vi "Alphanumeric_keyboard_new.vi"(0 "Str Refnum":refnum<vi>, 1 "Display Style":u32) -> (2 "New String":string, 3 "Previous String":string, 4 "Boolean":bool)   [LabVIEW 2022 SP3]
doc: "This VI takes the control reference for a digital numeric indicator and provides a calculator style keypad for number entry. The reference is double, but it only works for positive, integer values"
uses:
  <vilib>/Utility/miscctls.llb/LVPointTypeDef.ctl
panel:
  in  "SBR":bool
  in  "SBL":bool
  in  "CBR":bool
  in  "CBL":bool
  in  "RBR":bool
  in  "RBL":bool
  in  "Zero":bool
  in  "Percentage":bool
  in  "Space":bool
  in  "Dolor":bool
  in  "Plus":bool
  in  "@":bool
  in  "Under Score":bool
  in  "Has":bool
  in  "Star":bool
  in  "and":bool
  in  "Caps Lock":bool
  in  "Equal":bool
  in  "X":bool
  in  "Z":bool
  in  "C":bool
  in  "Backslash":bool
  in  "Slash":bool
  in  "M":bool
  in  "N":bool
  in  "B":bool
  in  "V":bool
  in  "Minus":bool
  in  "Colon":bool
  in  "S":bool
  in  "D":bool
  in  "A":bool
  in  "Semi Colon":bool
  in  "L":bool
  in  "K":bool
  in  "J":bool
  in  "H":bool
  in  "G":bool
  in  "F":bool
  in  "Comma":bool
  in  "W":bool
  in  "E":bool
  in  "Q":bool
  in  "P":bool
  in  "O":bool
  in  "I":bool
  in  "U":bool
  in  "Y":bool
  in  "T":bool
  in  "R":bool
  in  "Dot":bool
  in  "Enter Text":string
  in  "Enter":bool
  in  "Nine":bool
  in  "Eight":bool
  in  "Seven":bool
  in  "Six":bool
  in  "Five":bool
  in  "Four":bool
  in  "Three":bool
  in  "CLR":bool
  in  "BS":bool
  in  "Cancel":bool
  in  "Two":bool
  in  "One":bool
  out "String":string
  in  "Charactor\nLength":dbl
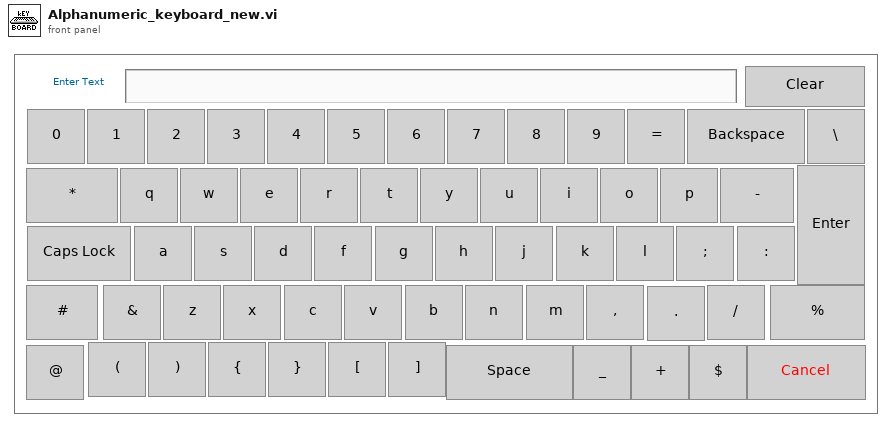
[diagram p1: front panel]
types:
  T1 = typedef "LVPointTypeDef.ctl" = cluster{"Horizontal":i16, "Vertical":i16}
  T2 = enum32{"Invalid", "Default", "Floating", "Floating/Auto-Hide", "Modal"}
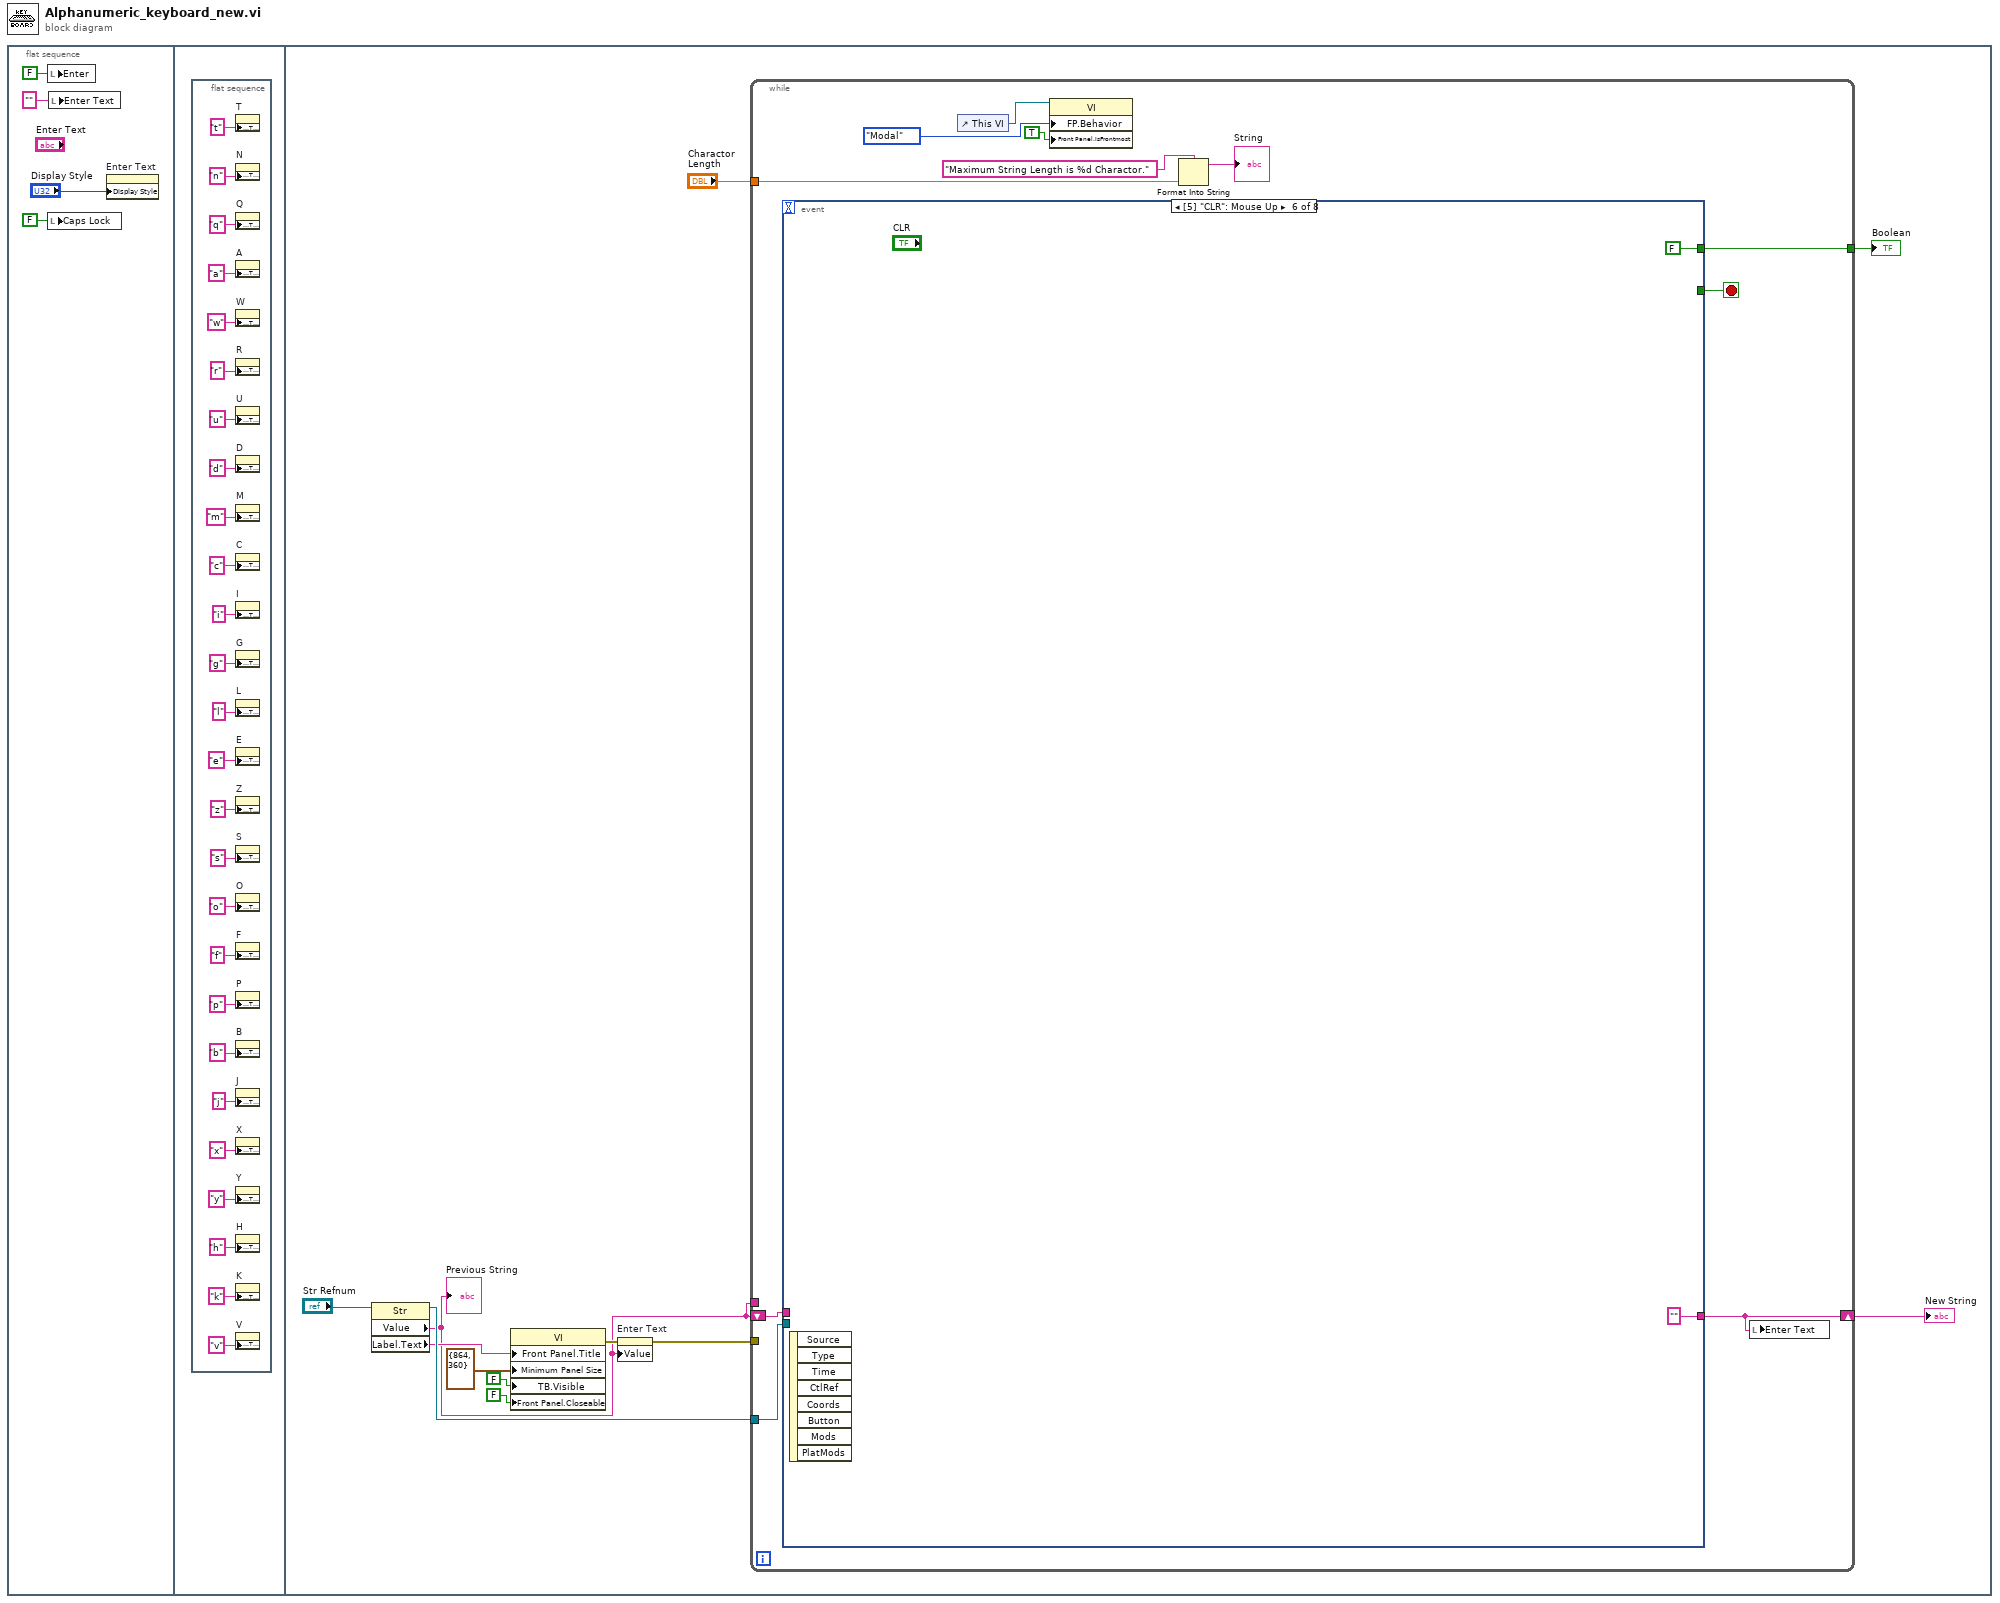
[diagram p0: block diagram]
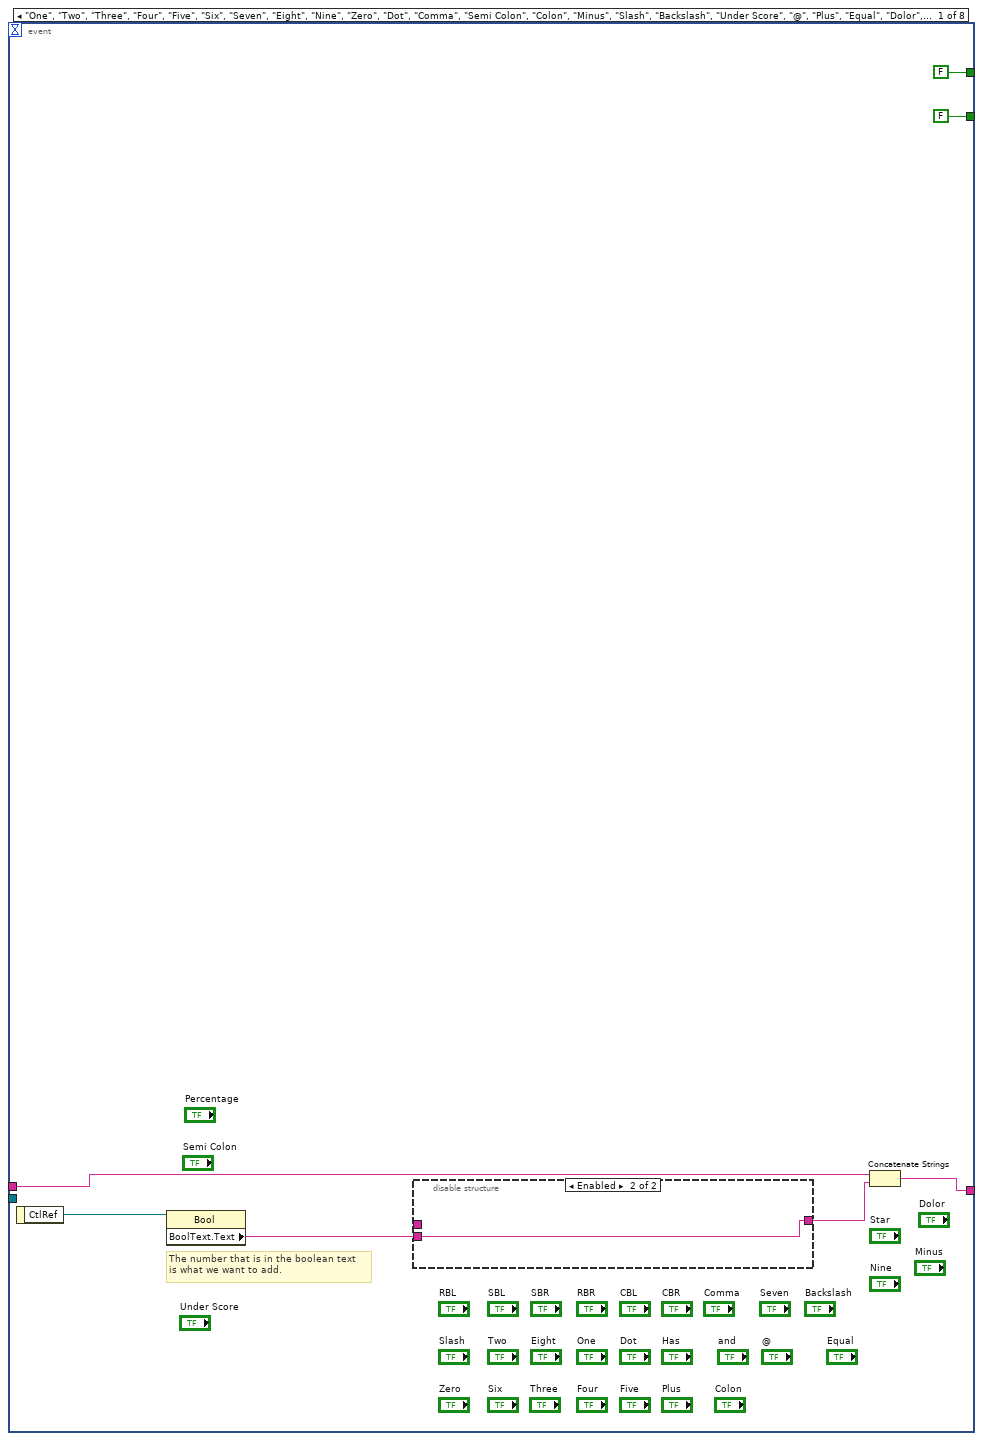
[diagram p2: hidden frame]
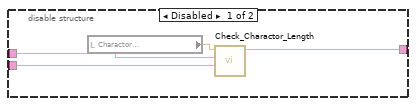
[diagram p3: hidden frame]
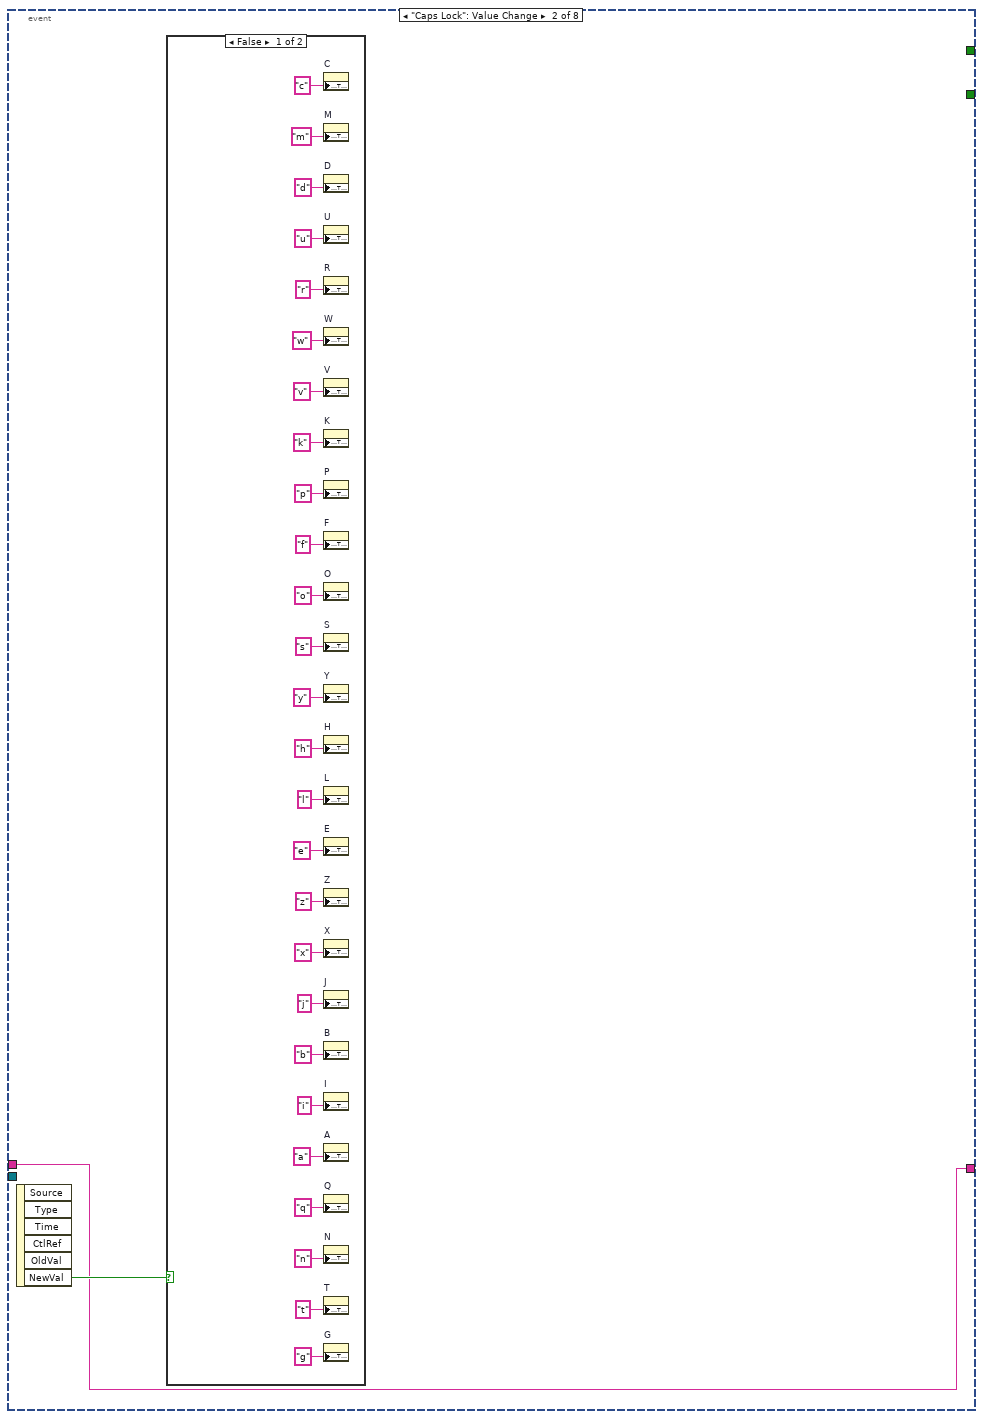
[diagram p4: hidden frame]
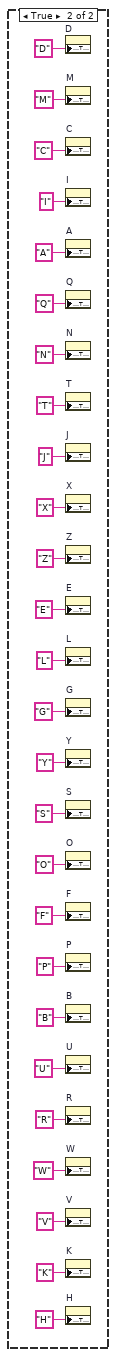
[diagram p5: hidden frame]
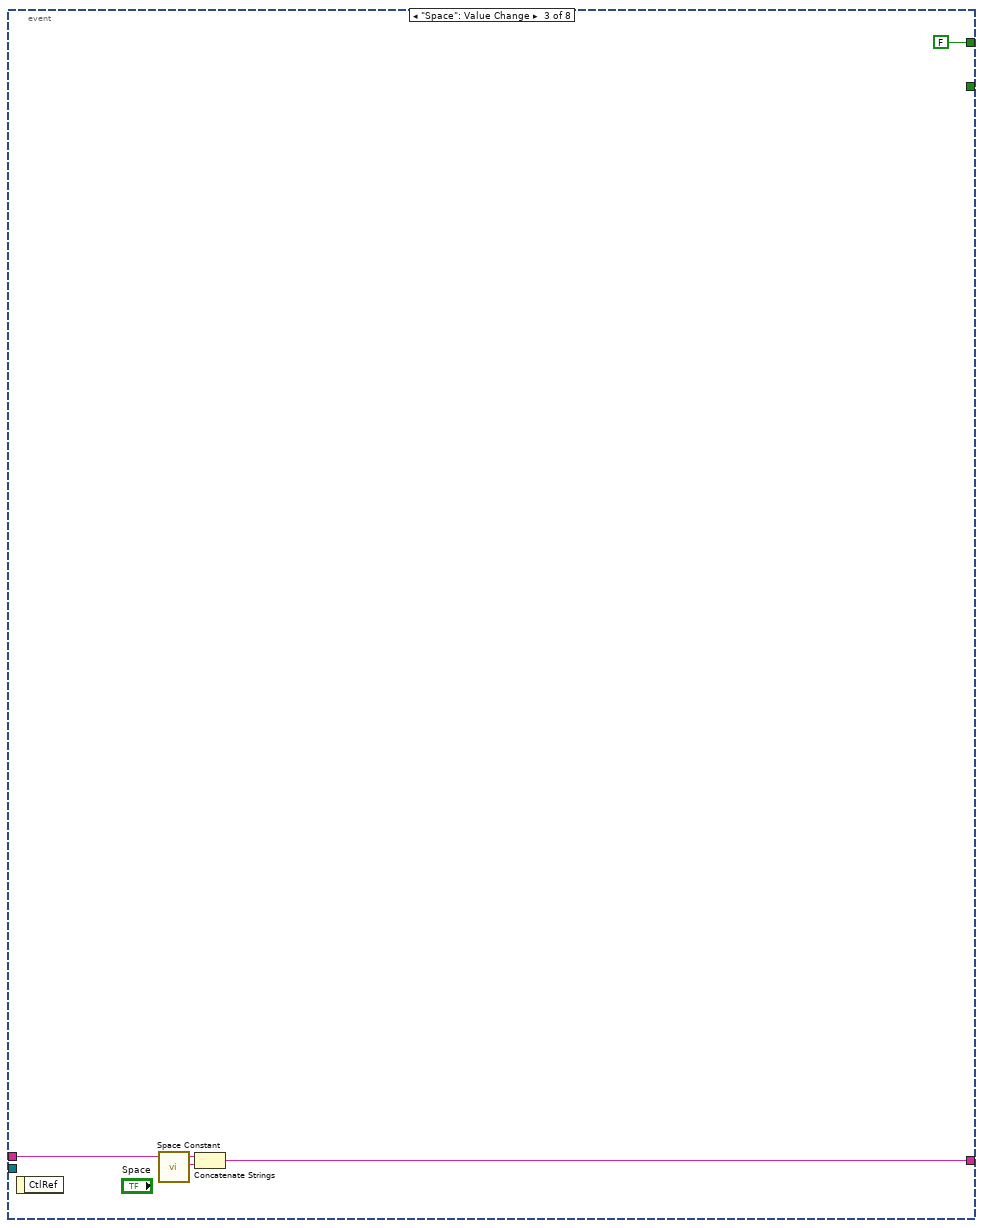
[diagram p6: hidden frame]
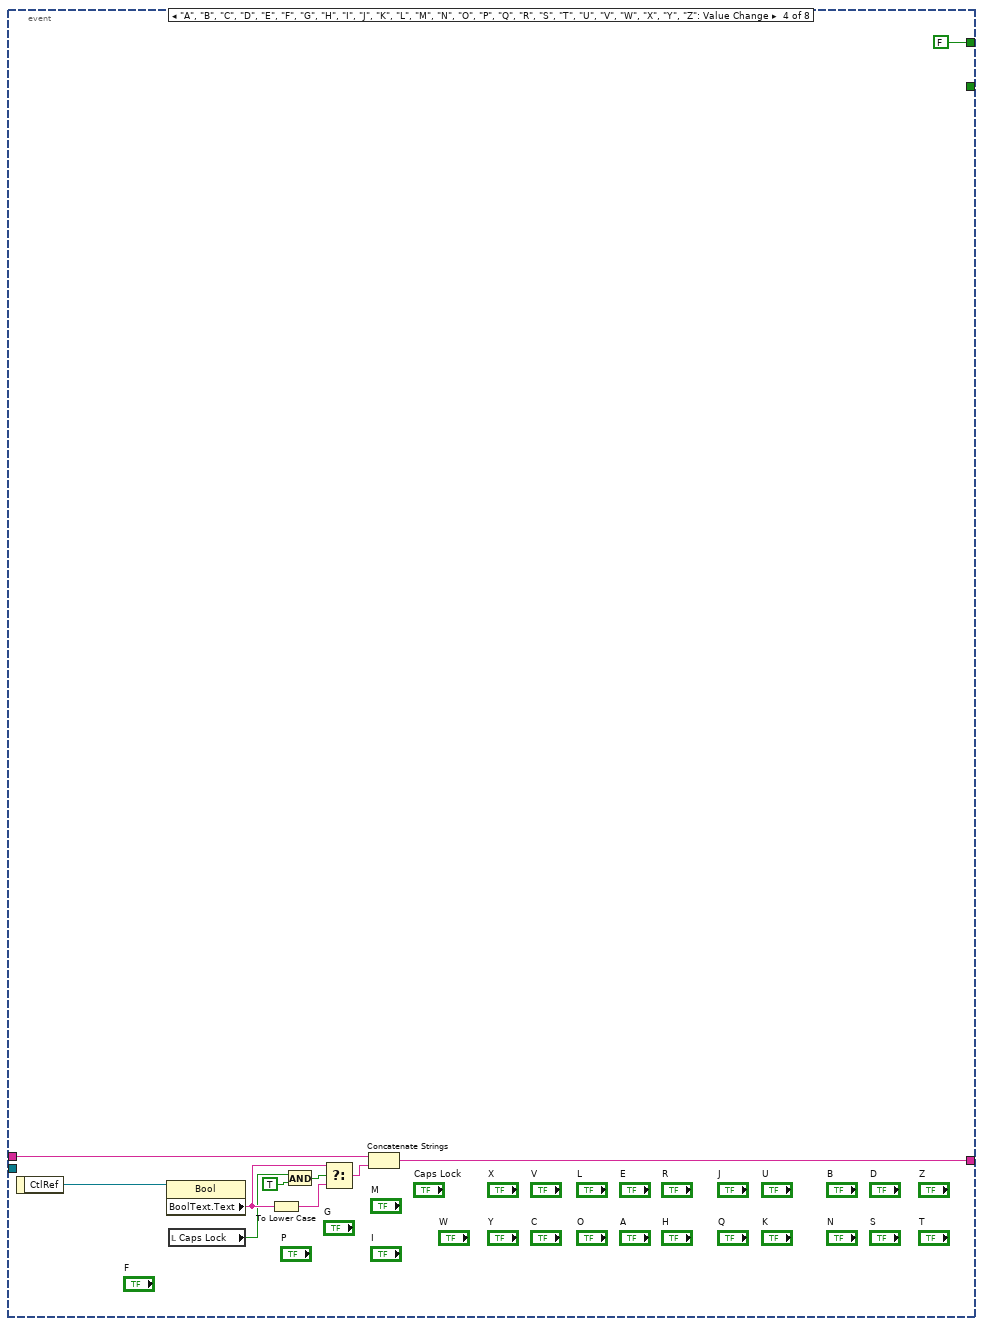
[diagram p7: hidden frame]
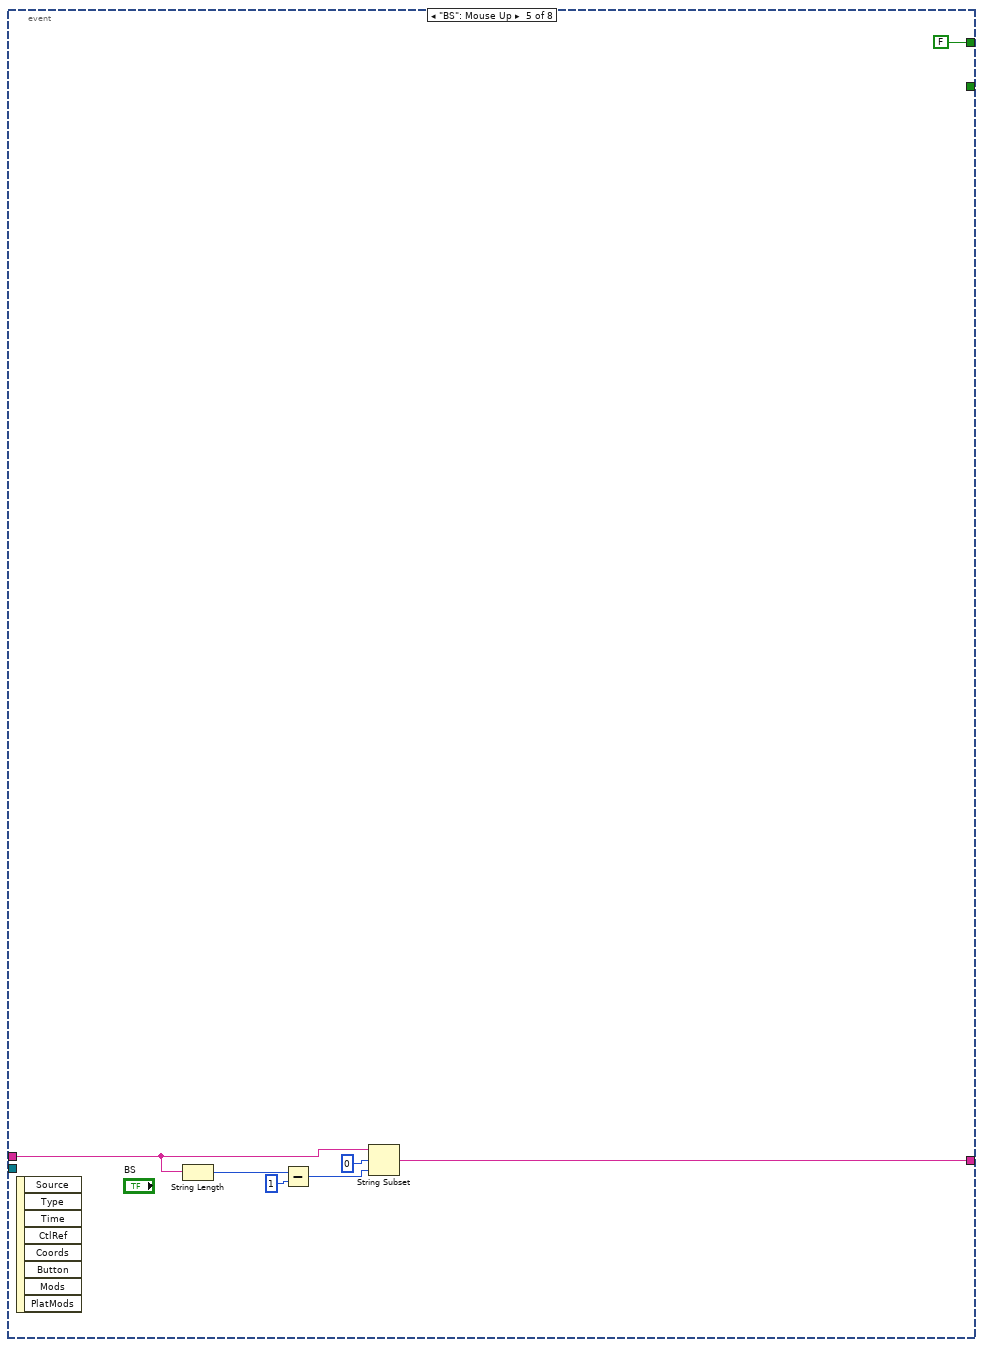
[diagram p8: hidden frame]
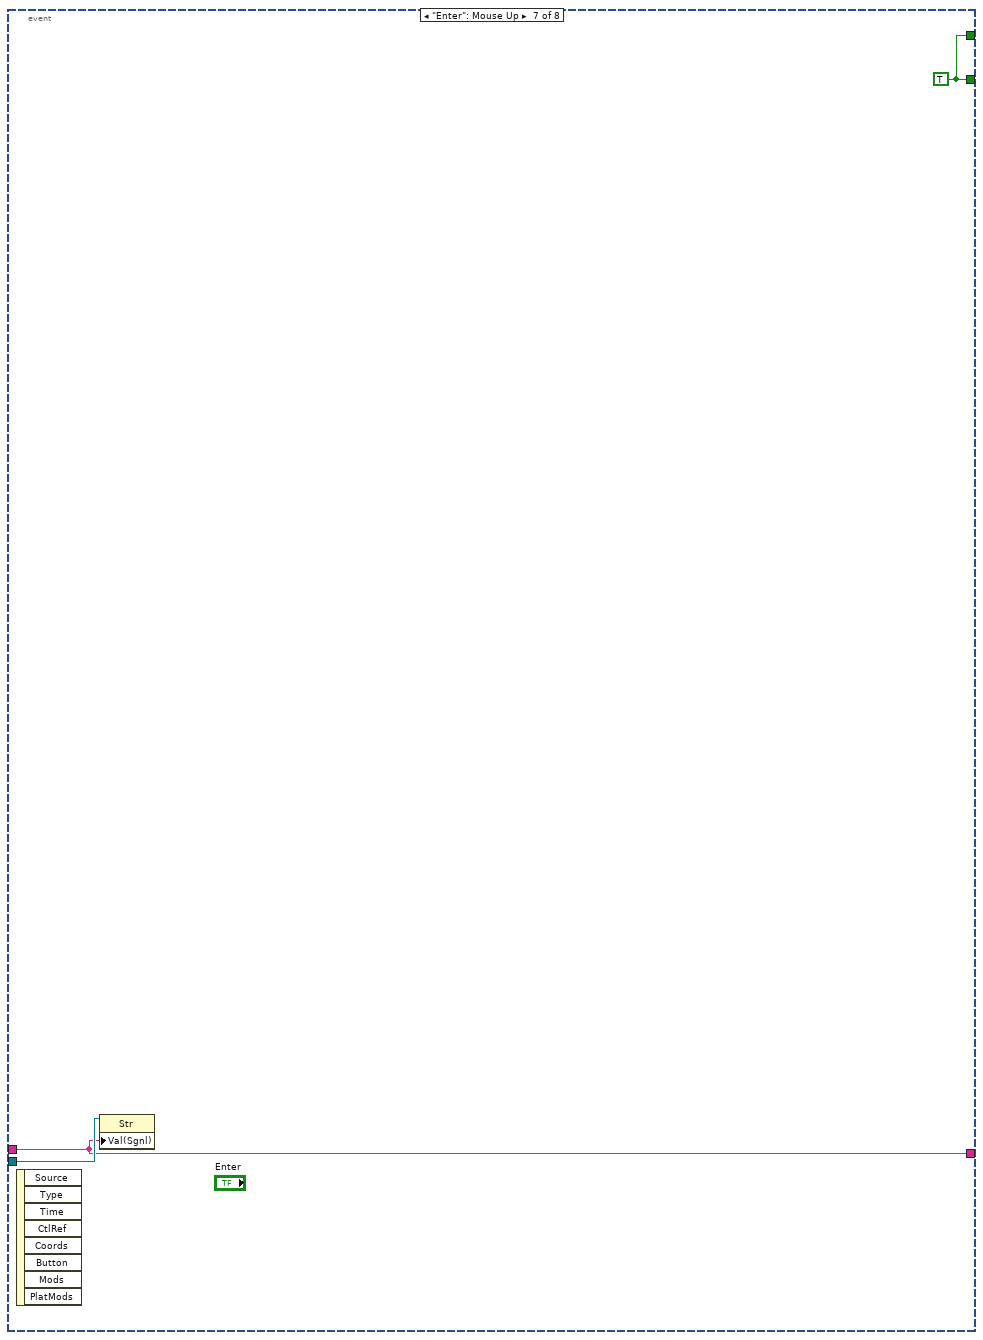
[diagram p9: hidden frame]
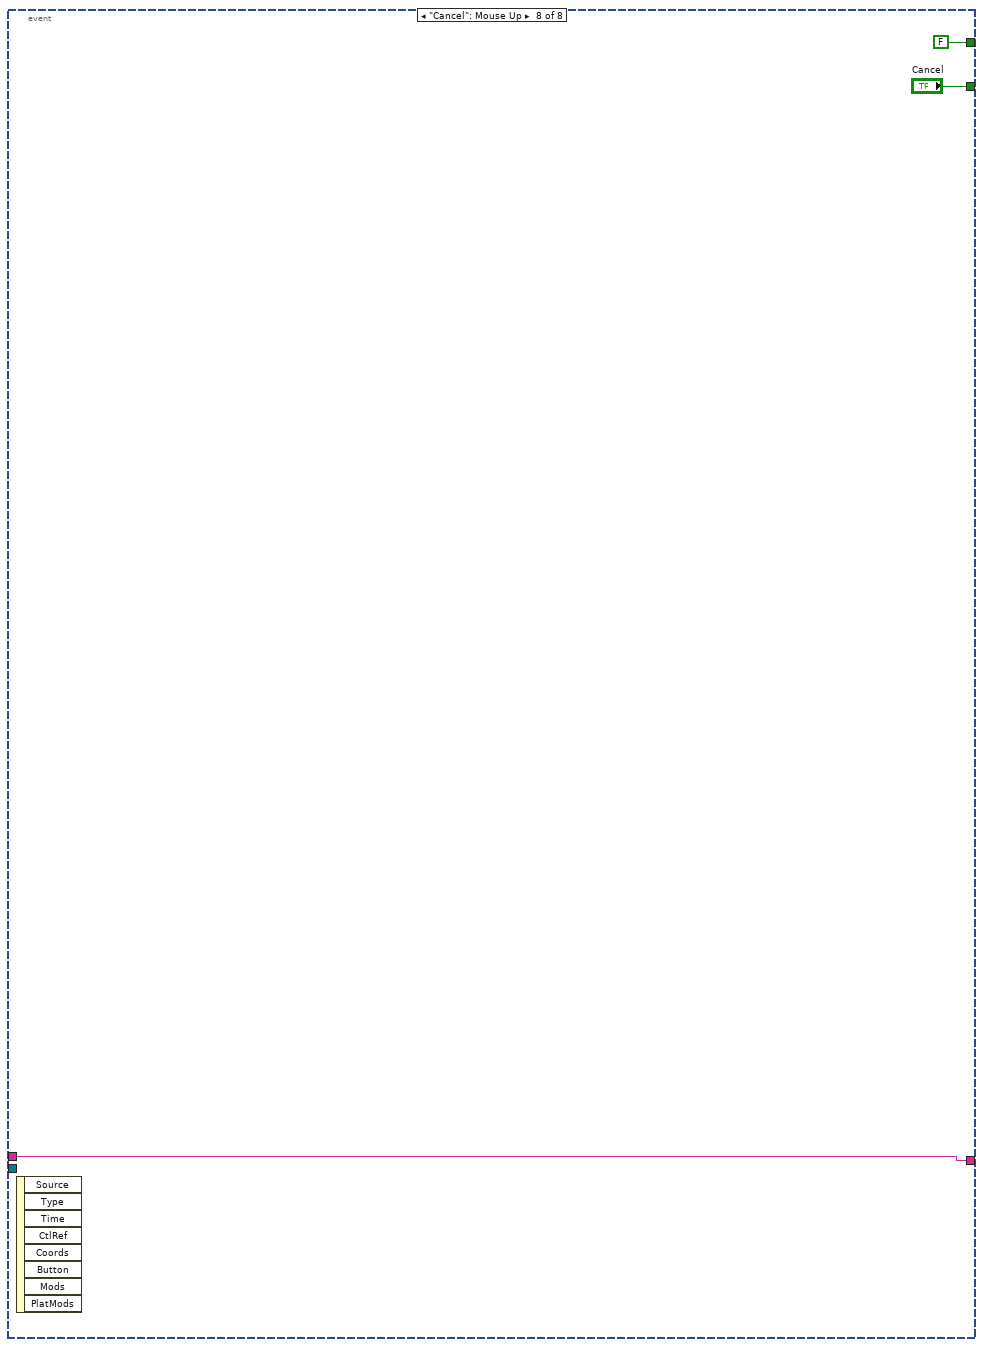
[diagram p10: hidden frame]
diagram:
  n1 = flat-sequence {
    frame #0 {
      n2 = local write "Enter"(FALSE ("Enter")) -> ()
      n3 = local write "Caps Lock"(FALSE ("Caps Lock")) -> ()
      n4 = local write "Enter Text"("" ("Enter Text")) -> ()
      n5 = property on="Enter Text" class="Str"("Display Style"="Display Style") -> ()  [unwired: 2 in, 2 out]
    }
    frame #1 {
      n6 = flat-sequence {
        frame #0 {
          n7 = property on="T" class="Bool"("BoolText.Text"="t" ("Boolean Text.Text")) -> ()  [unwired: 2 in, 2 out]
          n8 = property on="N" class="Bool"("BoolText.Text"="n" ("Boolean Text.Text")) -> ()  [unwired: 2 in, 2 out]
          n9 = property on="Q" class="Bool"("BoolText.Text"="q" ("Boolean Text.Text")) -> ()  [unwired: 2 in, 2 out]
          n10 = property on="A" class="Bool"("BoolText.Text"="a" ("Boolean Text.Text")) -> ()  [unwired: 2 in, 2 out]
          n11 = property on="W" class="Bool"("BoolText.Text"="w" ("Boolean Text.Text")) -> ()  [unwired: 2 in, 2 out]
          n12 = property on="R" class="Bool"("BoolText.Text"="r" ("Boolean Text.Text")) -> ()  [unwired: 2 in, 2 out]
          n13 = property on="U" class="Bool"("BoolText.Text"="u" ("Boolean Text.Text")) -> ()  [unwired: 2 in, 2 out]
          n14 = property on="D" class="Bool"("BoolText.Text"="d" ("Boolean Text.Text")) -> ()  [unwired: 2 in, 2 out]
          n15 = property on="M" class="Bool"("BoolText.Text"="m" ("Boolean Text.Text")) -> ()  [unwired: 2 in, 2 out]
          n16 = property on="C" class="Bool"("BoolText.Text"="c" ("Boolean Text.Text")) -> ()  [unwired: 2 in, 2 out]
          n17 = property on="I" class="Bool"("BoolText.Text"="i" ("Boolean Text.Text")) -> ()  [unwired: 2 in, 2 out]
          n18 = property on="G" class="Bool"("BoolText.Text"="g" ("Boolean Text.Text")) -> ()  [unwired: 2 in, 2 out]
          n19 = property on="L" class="Bool"("BoolText.Text"="l" ("Boolean Text.Text")) -> ()  [unwired: 2 in, 2 out]
          n20 = property on="E" class="Bool"("BoolText.Text"="e" ("Boolean Text.Text")) -> ()  [unwired: 2 in, 2 out]
          n21 = property on="Z" class="Bool"("BoolText.Text"="z" ("Boolean Text.Text")) -> ()  [unwired: 2 in, 2 out]
          n22 = property on="S" class="Bool"("BoolText.Text"="s" ("Boolean Text.Text")) -> ()  [unwired: 2 in, 2 out]
          n23 = property on="O" class="Bool"("BoolText.Text"="o" ("Boolean Text.Text")) -> ()  [unwired: 2 in, 2 out]
          n24 = property on="F" class="Bool"("BoolText.Text"="f" ("Boolean Text.Text")) -> ()  [unwired: 2 in, 2 out]
          n25 = property on="P" class="Bool"("BoolText.Text"="p" ("Boolean Text.Text")) -> ()  [unwired: 2 in, 2 out]
          n26 = property on="B" class="Bool"("BoolText.Text"="b" ("Boolean Text.Text")) -> ()  [unwired: 2 in, 2 out]
          n27 = property on="J" class="Bool"("BoolText.Text"="j" ("Boolean Text.Text")) -> ()  [unwired: 2 in, 2 out]
          n28 = property on="X" class="Bool"("BoolText.Text"="x" ("Boolean Text.Text")) -> ()  [unwired: 2 in, 2 out]
          n29 = property on="Y" class="Bool"("BoolText.Text"="y" ("Boolean Text.Text")) -> ()  [unwired: 2 in, 2 out]
          n30 = property on="H" class="Bool"("BoolText.Text"="h" ("Boolean Text.Text")) -> ()  [unwired: 2 in, 2 out]
          n31 = property on="K" class="Bool"("BoolText.Text"="k" ("Boolean Text.Text")) -> ()  [unwired: 2 in, 2 out]
          n32 = property on="V" class="Bool"("BoolText.Text"="v" ("Boolean Text.Text")) -> ()  [unwired: 2 in, 2 out]
        }
      }
    }
    frame #2 {
      n33 = property class="Str"(reference="Str Refnum") -> (reference out=w42:refnum<vi>, "Value"=w31:string, "Label.Text"=w41:string)  [unwired: 1 in, 1 out]
      "Previous String" <- w31
      n34 = property class="VI"("Front Panel.Title"=w41, "Minimum Panel Size"=T1 {"Horizontal"=864, "Vertical"=360} ("Front Panel Window:Minimum Size"), "TB.Visible"=FALSE ("Tool Bar:Visible"), "Front Panel.Closeable"=FALSE ("Front Panel Window:Resizable")) -> (error out=w32:errorcluster)  [unwired: 2 in, 1 out]
      n35 = property on="Enter Text" class="Str"(error in=w32, "Value"=w31) -> (error out=w40:errorcluster)  [unwired: 1 in, 1 out]
      n36 = while {
        tunnel: w42 -> [w52]
        tunnel: w40 -> [_]
        tunnel: "Charactor\nLength" -> [w51]
        tunnel: w31 -> [_]
        tunnel: [w48] -> w34
        shift-right: [w43] -> w33
        shift-left: w31 -> [w44]
        stop <- w53 stop-if-true
        n37 = event shown="[5] \"CLR\": Mouse Up" {
          selector: _ -> [_ _ _ _ _ _ _ _]
          dyn-events: _ -> [_ _ _ _ _ _ _ _]
          timeout: _ -> [_ _ _ _ _ _ _ _]
          tunnel: [FALSE _ _ _ _ _ w144 "Cancel"] -> w53
          tunnel: w52 -> [_ _ _ _ _ _ w145 _]
          tunnel: [FALSE ("Cancel") _ FALSE ("Cancel") FALSE ("Cancel") FALSE ("Cancel") FALSE ("Cancel") w144 FALSE ("Cancel")] -> w48
          tunnel: [w55 w66 w121 w126 w134 "" ("Enter Text") w143 w146] -> w43
          tunnel: w44 -> [w56 w66 w122 w125 w135 _ w143 w146]
          event "One", "Two", "Three", "Four", "Five", "Six", "Seven", "Eight", "Nine", "Zero", "Dot", "Comma", "Semi Colon", "Colon", "Minus", "Slash", "Backslash", "Under Score", "@", "Plus", "Equal", "Dolor", "Has", "and", "Star", "Percentage", "RBL", "RBR", "CBL", "CBR", "SBL", "SBR": Value Change {
            # "The number that is in the boolean text\nis what we want to add."
            n38 = event-data() -> ("CtlRef"=w60:refnum<vi>)  [unwired: 1 out]
            n39 = property class="Bool"(reference=w60) -> ("BoolText.Text"=w58:string)  [unwired: 1 in, 2 out]
            n40 = disable-structure shown="Enabled" {
              disable-tunnel: _ -> [w64 _]
              disable-tunnel: w58 -> [w63 w65]
              disable-tunnel: [w61 w65] -> w54
              frame Disabled {
                n41 = local read "Charactor\nLength"() -> (w62:dbl)
                n42 = call "Check_Charactor_Length.vi"("BoolText.Text"=w63, "New String"=w64, "Charactor\nLength"=w62) -> ("String"=w61:string)  [unwired: 8 in]
              }
              frame Enabled {
              }
            }
            n43 = Concatenate Strings(w56, w54) -> (w55:string)
          }
          event "Caps Lock": Value Change {
            n44 = event-data() -> ("NewVal"=w67:bool)  [unwired: 6 out]
            n45 = case shown="False" w67 {
              frame False {
                n46 = property on="C" class="Bool"("BoolText.Text"="c" ("Boolean Text.Text")) -> ()  [unwired: 2 in, 2 out]
                n47 = property on="M" class="Bool"("BoolText.Text"="m" ("Boolean Text.Text")) -> ()  [unwired: 2 in, 2 out]
                n48 = property on="D" class="Bool"("BoolText.Text"="d" ("Boolean Text.Text")) -> ()  [unwired: 2 in, 2 out]
                n49 = property on="U" class="Bool"("BoolText.Text"="u" ("Boolean Text.Text")) -> ()  [unwired: 2 in, 2 out]
                n50 = property on="R" class="Bool"("BoolText.Text"="r" ("Boolean Text.Text")) -> ()  [unwired: 2 in, 2 out]
                n51 = property on="W" class="Bool"("BoolText.Text"="w" ("Boolean Text.Text")) -> ()  [unwired: 2 in, 2 out]
                n52 = property on="V" class="Bool"("BoolText.Text"="v" ("Boolean Text.Text")) -> ()  [unwired: 2 in, 2 out]
                n53 = property on="K" class="Bool"("BoolText.Text"="k" ("Boolean Text.Text")) -> ()  [unwired: 2 in, 2 out]
                n54 = property on="P" class="Bool"("BoolText.Text"="p" ("Boolean Text.Text")) -> ()  [unwired: 2 in, 2 out]
                n55 = property on="F" class="Bool"("BoolText.Text"="f" ("Boolean Text.Text")) -> ()  [unwired: 2 in, 2 out]
                n56 = property on="O" class="Bool"("BoolText.Text"="o" ("Boolean Text.Text")) -> ()  [unwired: 2 in, 2 out]
                n57 = property on="S" class="Bool"("BoolText.Text"="s" ("Boolean Text.Text")) -> ()  [unwired: 2 in, 2 out]
                n58 = property on="Y" class="Bool"("BoolText.Text"="y" ("Boolean Text.Text")) -> ()  [unwired: 2 in, 2 out]
                n59 = property on="H" class="Bool"("BoolText.Text"="h" ("Boolean Text.Text")) -> ()  [unwired: 2 in, 2 out]
                n60 = property on="L" class="Bool"("BoolText.Text"="l" ("Boolean Text.Text")) -> ()  [unwired: 2 in, 2 out]
                n61 = property on="E" class="Bool"("BoolText.Text"="e" ("Boolean Text.Text")) -> ()  [unwired: 2 in, 2 out]
                n62 = property on="Z" class="Bool"("BoolText.Text"="z" ("Boolean Text.Text")) -> ()  [unwired: 2 in, 2 out]
                n63 = property on="X" class="Bool"("BoolText.Text"="x" ("Boolean Text.Text")) -> ()  [unwired: 2 in, 2 out]
                n64 = property on="J" class="Bool"("BoolText.Text"="j" ("Boolean Text.Text")) -> ()  [unwired: 2 in, 2 out]
                n65 = property on="B" class="Bool"("BoolText.Text"="b" ("Boolean Text.Text")) -> ()  [unwired: 2 in, 2 out]
                n66 = property on="I" class="Bool"("BoolText.Text"="i" ("Boolean Text.Text")) -> ()  [unwired: 2 in, 2 out]
                n67 = property on="A" class="Bool"("BoolText.Text"="a" ("Boolean Text.Text")) -> ()  [unwired: 2 in, 2 out]
                n68 = property on="Q" class="Bool"("BoolText.Text"="q" ("Boolean Text.Text")) -> ()  [unwired: 2 in, 2 out]
                n69 = property on="N" class="Bool"("BoolText.Text"="n" ("Boolean Text.Text")) -> ()  [unwired: 2 in, 2 out]
                n70 = property on="T" class="Bool"("BoolText.Text"="t" ("Boolean Text.Text")) -> ()  [unwired: 2 in, 2 out]
                n71 = property on="G" class="Bool"("BoolText.Text"="g" ("Boolean Text.Text")) -> ()  [unwired: 2 in, 2 out]
              }
              frame True {
                n72 = property on="D" class="Bool"("BoolText.Text"="D" ("Boolean Text.Text")) -> ()  [unwired: 2 in, 2 out]
                n73 = property on="M" class="Bool"("BoolText.Text"="M" ("Boolean Text.Text")) -> ()  [unwired: 2 in, 2 out]
                n74 = property on="C" class="Bool"("BoolText.Text"="C" ("Boolean Text.Text")) -> ()  [unwired: 2 in, 2 out]
                n75 = property on="I" class="Bool"("BoolText.Text"="I" ("Boolean Text.Text")) -> ()  [unwired: 2 in, 2 out]
                n76 = property on="A" class="Bool"("BoolText.Text"="A" ("Boolean Text.Text")) -> ()  [unwired: 2 in, 2 out]
                n77 = property on="Q" class="Bool"("BoolText.Text"="Q" ("Boolean Text.Text")) -> ()  [unwired: 2 in, 2 out]
                n78 = property on="N" class="Bool"("BoolText.Text"="N" ("Boolean Text.Text")) -> ()  [unwired: 2 in, 2 out]
                n79 = property on="T" class="Bool"("BoolText.Text"="T" ("Boolean Text.Text")) -> ()  [unwired: 2 in, 2 out]
                n80 = property on="J" class="Bool"("BoolText.Text"="J" ("Boolean Text.Text")) -> ()  [unwired: 2 in, 2 out]
                n81 = property on="X" class="Bool"("BoolText.Text"="X" ("Boolean Text.Text")) -> ()  [unwired: 2 in, 2 out]
                n82 = property on="Z" class="Bool"("BoolText.Text"="Z" ("Boolean Text.Text")) -> ()  [unwired: 2 in, 2 out]
                n83 = property on="E" class="Bool"("BoolText.Text"="E" ("Boolean Text.Text")) -> ()  [unwired: 2 in, 2 out]
                n84 = property on="L" class="Bool"("BoolText.Text"="L" ("Boolean Text.Text")) -> ()  [unwired: 2 in, 2 out]
                n85 = property on="G" class="Bool"("BoolText.Text"="G" ("Boolean Text.Text")) -> ()  [unwired: 2 in, 2 out]
                n86 = property on="Y" class="Bool"("BoolText.Text"="Y" ("Boolean Text.Text")) -> ()  [unwired: 2 in, 2 out]
                n87 = property on="S" class="Bool"("BoolText.Text"="S" ("Boolean Text.Text")) -> ()  [unwired: 2 in, 2 out]
                n88 = property on="O" class="Bool"("BoolText.Text"="O" ("Boolean Text.Text")) -> ()  [unwired: 2 in, 2 out]
                n89 = property on="F" class="Bool"("BoolText.Text"="F" ("Boolean Text.Text")) -> ()  [unwired: 2 in, 2 out]
                n90 = property on="P" class="Bool"("BoolText.Text"="P" ("Boolean Text.Text")) -> ()  [unwired: 2 in, 2 out]
                n91 = property on="B" class="Bool"("BoolText.Text"="B" ("Boolean Text.Text")) -> ()  [unwired: 2 in, 2 out]
                n92 = property on="U" class="Bool"("BoolText.Text"="U" ("Boolean Text.Text")) -> ()  [unwired: 2 in, 2 out]
                n93 = property on="R" class="Bool"("BoolText.Text"="R" ("Boolean Text.Text")) -> ()  [unwired: 2 in, 2 out]
                n94 = property on="W" class="Bool"("BoolText.Text"="W" ("Boolean Text.Text")) -> ()  [unwired: 2 in, 2 out]
                n95 = property on="V" class="Bool"("BoolText.Text"="V" ("Boolean Text.Text")) -> ()  [unwired: 2 in, 2 out]
                n96 = property on="K" class="Bool"("BoolText.Text"="K" ("Boolean Text.Text")) -> ()  [unwired: 2 in, 2 out]
                n97 = property on="H" class="Bool"("BoolText.Text"="H" ("Boolean Text.Text")) -> ()  [unwired: 2 in, 2 out]
              }
            }
          }
          event "Space": Value Change {
            n98 = event-data() -> ()  [unwired: 2 out]
            n99 = call <vilib>:"Space Constant.vi"() -> ("String"=w120:string)
            n100 = Concatenate Strings(w122, w120) -> (w121:string)
          }
          event "A", "B", "C", "D", "E", "F", "G", "H", "I", "J", "K", "L", "M", "N", "O", "P", "Q", "R", "S", "T", "U", "V", "W", "X", "Y", "Z": Value Change {
            n101 = event-data() -> ("CtlRef"=w133:refnum<vi>)  [unwired: 1 out]
            n102 = property class="Bool"(reference=w133) -> ("BoolText.Text"=w130:string)  [unwired: 1 in, 2 out]
            n103 = local read "Caps Lock"() -> (w128:bool)
            n104 = To Lower Case(string=w130) -> (all lower case string=w129:string)
            n105 = And(x=w128, y=TRUE) -> (x .and. y?=w131:bool)
            n106 = Select(t=w130, s=w131, f=w129) -> (s? t:f=w124:string)
            n107 = Concatenate Strings(w125, w124) -> (w126:string)
          }
          event "BS": Mouse Up {
            n108 = event-data() -> ()  [unwired: 9 out]
            n109 = String Length(string=w135) -> (length=w139:i32)
            n110 = Subtract(x=w139, y=1) -> (x-y=w138:i32)
            n111 = String Subset(string=w135, offset (0)=0, length (rest)=w138) -> (substring=w134:string)
          }
          event "CLR": Mouse Up {
            n112 = event-data() -> ()  [unwired: 9 out]
          }
          event "Enter": Mouse Up {
            w144 = TRUE ("Cancel")
            n113 = event-data() -> ()  [unwired: 9 out]
            n114 = property class="Str"(reference=w145, "Val(Sgnl)"=w143) -> ()  [unwired: 1 in, 2 out]
          }
          event "Cancel": Mouse Up {
            n115 = event-data() -> ()  [unwired: 9 out]
          }
        }
        n116 = control-ref of="This VI"() -> (w45:refnum<vi>)
        n117 = property class="VI"(reference=w45, "FP.Behavior"=T2."Modal" ("Front Panel Window:Behavior"), "Front Panel.IsFrontmost"=TRUE ("Front Panel Window:Is Frontmost")) -> ()  [unwired: 1 in, 2 out]
        n118 = Format Into String(format string="Maximum String Length is %d Charactor.", w51) -> (resulting string=→"String":string)  [unwired: 2 in, 1 out]
        n119 = local write "Enter Text"(w43) -> ()
      }
      "New String" <- w33
      "Boolean" <- w34
    }
  }
